vi "Remove Custom Device.vi"(8 "error in (no error)":errorcluster, 11 "CD Ref":T1 format="%.0x") -> (0 "error out":errorcluster)   [LabVIEW 2017, in "Switch Scripting.lvlib"]
uses:
  Switch Scripting.lvlib
  <vilib>/NI Veristand/Custom Device API/Custom Device Item Ref.ctl
  NationalInstruments.VeriStand.SystemDefinitionAPI
  <vilib>/NI VeriStand/Custom Device API/Custom Device API.lvlib
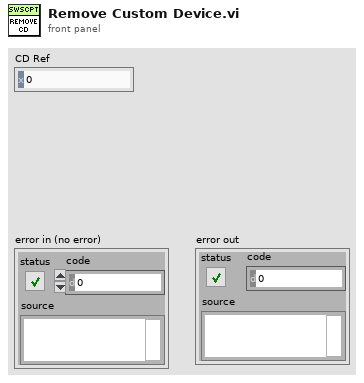
[diagram p1: front panel]
types:
  T1 = typedef "Custom Device API.lvlib/Custom Device Item Ref.ctl" = u64
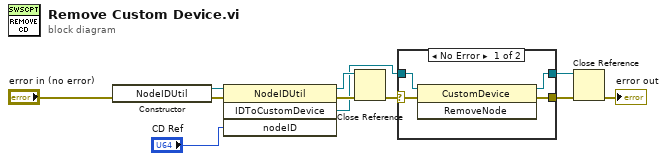
[diagram p0: block diagram]
diagram:
  n1 = constructor class="NodeIDUtil"(error in="error in (no error)") -> (reference out=w7:refnum<k24>, error out=w8:errorcluster)  [unwired: 2 in, 1 out]
  n2 = invoke class="NodeIDUtil" method="IDToCustomDevice"(reference=w7, error in=w8, "nodeID"="CD Ref") -> (reference out=w5:refnum<k24>, error out=w6:errorcluster, "IDToCustomDevice"=w3:refnum<k24>)  [unwired: 1 in, 1 out]
  n3 = Close Reference(reference=w5, error in (no error)=w6) -> (error out=w1:errorcluster)
  n4 = case shown="No Error" w1 {
    selector: w1 -> [w14 w17]
    tunnel: w3 -> [w15 w16]
    tunnel: [w13 w16] -> w11
    tunnel: [w12 w17] -> w10
    frame No Error {
      n5 = invoke class="CustomDevice" method="RemoveNode"(reference=w15, error in=w14) -> (reference out=w13:refnum<k24>, error out=w12:errorcluster)  [unwired: 1 in, 1 out]
    }
    frame Error {
    }
  }
  n6 = Close Reference(reference=w11, error in (no error)=w10) -> (error out=→"error out":errorcluster)
